vi "Dashboard Main.vi"() -> ()   [LabVIEW 2017]
uses:
  <vilib>/Rock Robotics/Network Tables/NT Read Numeric Array.vi
  <vilib>/Rock Robotics/Network Tables/NT Read Number.vi
  <vilib>/Rock Robotics/Network Tables/NT Write Boolean.vi
panel:
  out "Camera Info":cluster{"Mbps LED":bool, "Mbps":dbl, "fps":dbl} {"fps" format="%#.1g"; "Mbps" format="%#.1g"}
  in  "Camera Settings":T1={"Frame Rate"=30, "Compression"=30, "Size"=1, "DB Camera Config"=FALSE} {"Frame Rate" scale=1.0..30.0; "Compression" scale=100.0..-1.0; "Size" items=["640x480", "320x240", "160x120"]}
  in  "TCP":refnum<k5>
  out "Robot IP":string
  in  "Dashboard Tab":enum32{"Drive", "Basic", "Custom", "Variables"}(tab)
  out "Accel mins":dbl[](array[numeric])
  in  "Boolean":bool
  out "AvgY":dbl
  out "AvgX":dbl
  out "Accel maxs":dbl[](array[numeric])
  out "Accels":dbl[](array[numeric])
  out "Gyro rate":dbl
  out "Gyro":dbl
  in  "Select Auto":string(combo)="Select Autonomous ..."
  out "NT Connection":bool
  out "MotorChart R":cluster{"Numeric":dbl, "Numeric":dbl}(graph)
  out "MotorChart L":cluster{"Numeric":dbl, "Numeric":dbl}(graph)
  out "MotorSliders R":cluster{"MotorSlide1":dbl, "MotorSlide2":dbl} {"MotorSlide2" scale=-1.0..1.0 scale format="%#_2e"; "MotorSlide1" scale=-1.0..1.0 scale format="%#_2e"}
  out "MotorSliders L":cluster{"MotorSlide1":dbl, "MotorSlide2":dbl} {"MotorSlide2" scale=-1.0..1.0 scale format="%#_2e"; "MotorSlide1" scale=-1.0..1.0 scale format="%#_2e"}
  out "JS1 Z":dbl(slide) scale=-1.0..1.0 scale format="%#_2e"
  out "JS1 Graph":cluster{"X":dbl, "Y":dbl}[](graph)
  out "JS1 Buttons":T2
  out "JS2 Z":dbl(slide) scale=-1.0..1.0 scale format="%#_2e"
  out "JS2 Graph":cluster{"X":dbl, "Y":dbl}[](graph)
  out "JS2 Buttons":T2
  out "Mode":T3(ring)=enum."Auto Disabled"
  in  "DB/String 9":string
  in  "DB/String 8":string
  in  "DB/String 7":string
  in  "DB/String 6":string
  in  "DB/String 5":string
  in  "DB/String 4":string
  in  "DB/String 3":string
  in  "DB/String 2":string
  in  "DB/String 1":string
  in  "DB/String 0":string
  in  "DB/Slider 0":dbl(slide) scale=0.0..5.0
  in  "DB/Slider 1":dbl(slide) scale=0.0..5.0
  in  "DB/Slider 2":dbl(slide) scale=0.0..5.0
  in  "DB/Slider 3":dbl(slide) scale=0.0..5.0
  out "DB/LED 3":bool
  out "DB/LED 2":bool
  out "DB/LED 1":bool
  out "DB/LED 0":bool
  in  "DB/Button 3":bool
  in  "DB/Button 2":bool
  in  "DB/Button 1":bool
  in  "DB/Button 0":bool caption="New Name"
  out "Tree":string(tree)
  out "Camera Image":T4(plugin-control)
  out "Background":bool
  in  "Camera Name":string(combo)="No Camera Selection"
  # "HW"
  # "Joysticks"
  # "Drive Motors"
  # "Front"
  # "Right"
  # "Left"
  # "Back"
  # "This tab is a great place for autonomous settings and robot-specific values.\nPlace controls and indicators inside this tab and match name to\nDashboard Variables on robot. You can also delete this comment."
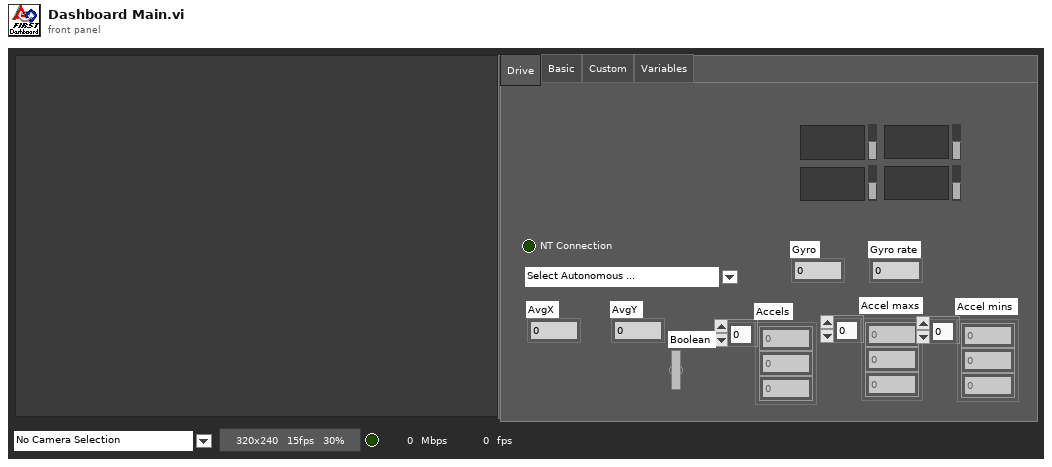
[diagram p1: front panel]
types:
  T1 = cluster{"Frame Rate":i32, "Compression":i32, "Size":u16, "DB Camera Config":bool}
  T2 = cluster{bool, bool, bool, bool, bool, bool, bool, bool, bool, bool, bool, bool}
  T3 = enum8{"Tele-Op Disabled", "Tele-Op Enabled", "Auto Disabled", "Auto Enabled", "Test Disabled", "Test Enabled", "Disconnected", "No Code", "E-Stop"}
  T4 = typedef "IMAQ Image.ctl" = refnum<image>
  T5 = cluster{"Save Path":path, "Interval (s)":dbl, "Keep":i32}
  T6 = typedef "Image Type" = u32
  T7 = cluster{"Camera Image":refnum<vi>, "Dashboard Tab":refnum<vi>, "Background":refnum<vi>, "Tree":refnum<vi>, "Camera Settings":refnum<vi>, "Camera Name":refnum<vi>, "Camera Info":refnum<vi>}
  T8 = cluster{"Error Strings":string, "Disable Counts":cluster{u16, u16}, "Rail Faults":cluster{u16, u16, u16}, "Robot IP":string, "DB Mode":u8, "Event Info":cluster{"Name":string, "Type":u8, "Number":u16, "Replay":u8}}
  T9 = cluster{"Storage":cluster{"Disk Free":u64, "RAM Block":u32, "RAM free":u32}, "CPU Utilization":cluster{"CPU % ISR":sgl, "CPU % Time Crit":sgl, "CPU % Timed Str":sgl, "CPU % High":sgl, "CPU % Above":sgl, "CPU % Normal":sgl, "CPU % Low":sgl}, "CAN":cluster{"% Bus Utilization":sgl, "Bus Off Cnt":u32, "TX_FIFO Full Cnt":u32, "Receive Error Cnt":u8, "Transmit Error Cnt":u8}, "HID":cluster{"HID Outputs":u32, "Rumble Low":u16, "Rumble High":u16}[]}
  T10 = cluster{"Status bits":cluster{"Test Mode":bool, "Autonomous":bool, "Enabled":bool, "Code Start":bool, "Brownout":bool, "Reserved 2":bool, "Reserved 3":bool, "E-Stop":bool}, "Code Trace":cluster{"Disabled":bool, "TeleOp":bool, "Auto":bool, "Test":bool}, "Controller Type":enum16{"unknown", "cRIO", "roboRio"}, "Code?":enum16{"unknown", "noCode", "code"}, "Battery V":dbl}
  T11 = cluster{"Control Bits":cluster{"TestMode":bool, "Autonomous":bool, "Enabled":bool, "FMS Present":bool, bool, bool, bool, "E-Stop":bool}, "Team Station ":u8, "Countdown":sgl, "Joystick Values":cluster{"Axes":dbl[], "Buttons":bool[], "POVs":i16[]}[]}
  T12 = cluster{"Axes":dbl[], "Buttons":bool[], "POVs":i16[]}[]
  T13 = cluster{"Axes":dbl[], "Buttons":bool[], "POVs":i16[]}
  T14 = cluster{"Buttons[0]":bool, "Buttons[1]":bool, "Buttons[2]":bool, "Buttons[3]":bool, "Buttons[4]":bool, "Buttons[5]":bool, "Buttons[6]":bool, "Buttons[7]":bool, "Buttons[8]":bool, "Buttons[9]":bool, "Buttons[10]":bool, "Buttons[11]":bool}
  T15 = cluster{"Shift":bool, "Ctrl":bool, "Alt":bool, "Cmd":bool, "Opt":bool}
  T16 = cluster{"Camera Name":string, "Camera File Name":string, "Saved DB Images Info":cluster{"Save Path":path, "Interval (s)":dbl, "Keep":i32}}
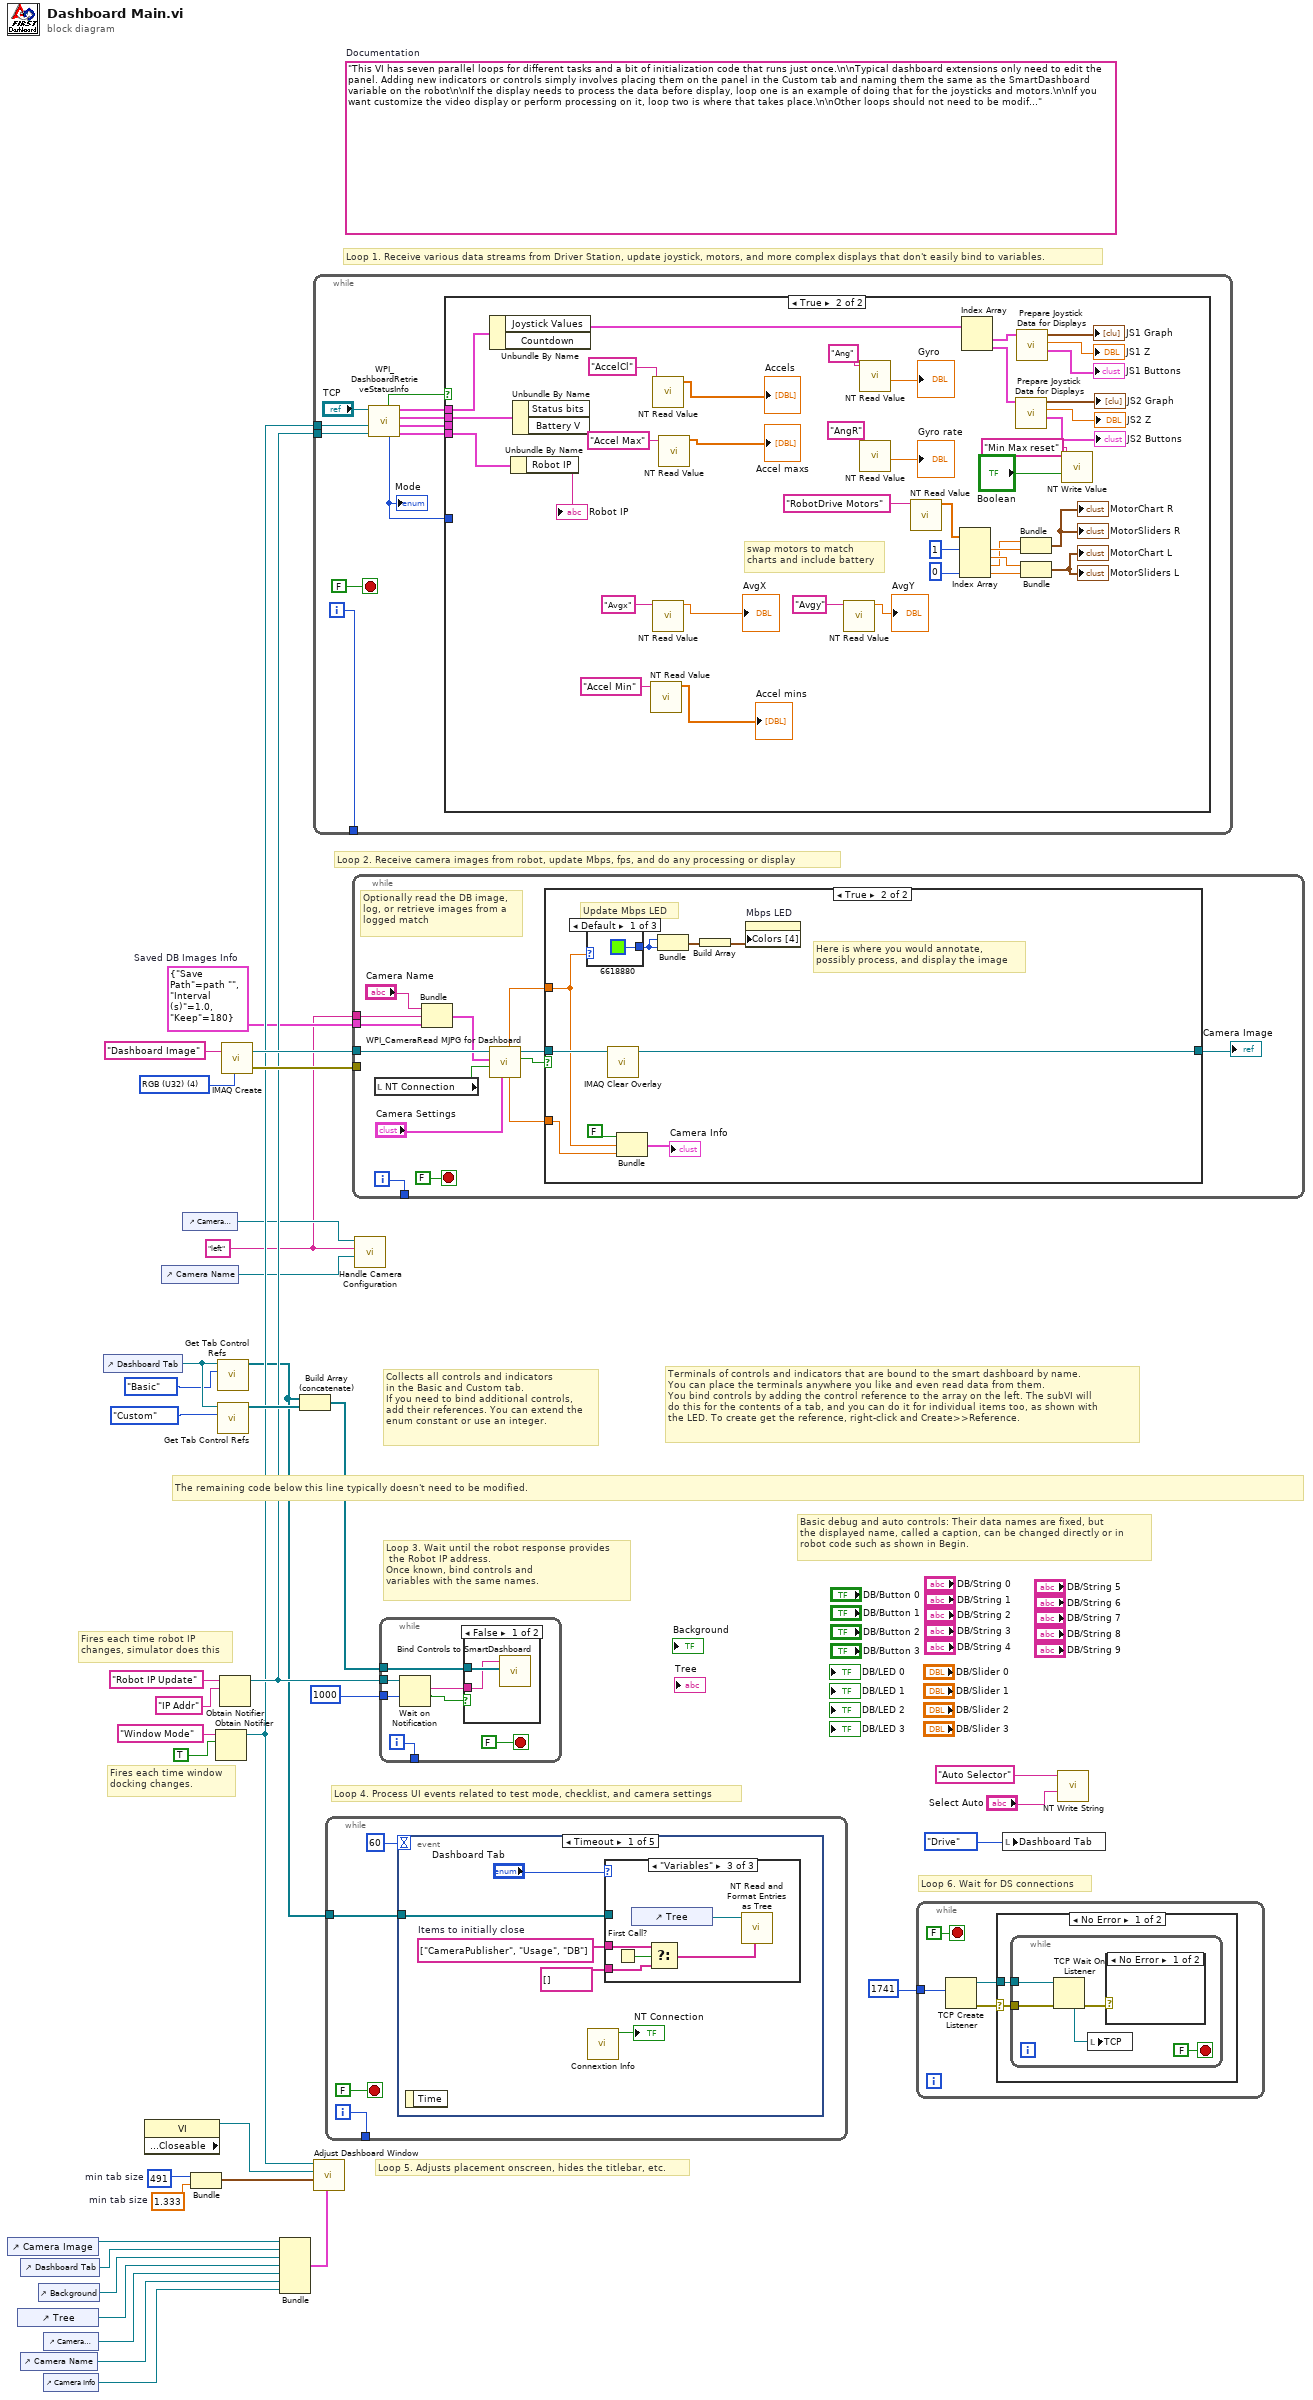
[diagram p0: block diagram]
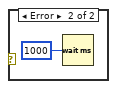
[diagram p2: hidden frame]
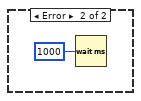
[diagram p3: hidden frame]
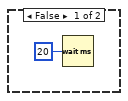
[diagram p4: hidden frame]
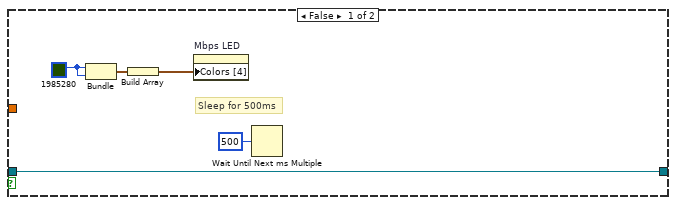
[diagram p6: hidden frame]
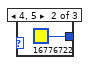
[diagram p7: hidden frame]
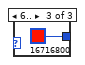
[diagram p8: hidden frame]
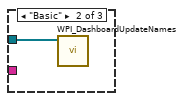
[diagram p10: hidden frame]
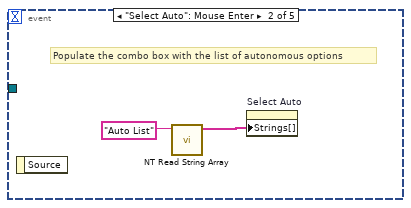
[diagram p11: hidden frame]
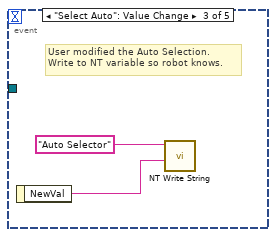
[diagram p12: hidden frame]
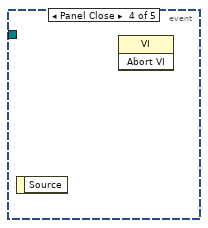
[diagram p13: hidden frame]
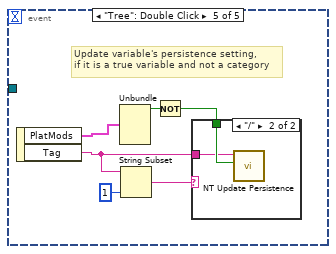
[diagram p14: hidden frame]
diagram:
  w1 = "left" ("Camera File Name")
  w2 = T5 {"Save Path"=path "", "Interval (s)"=1.0, "Keep"=180}  # Saved DB Images Info
  w22 = 491  # min tab size
  w21 = 1.333  # min tab size
  (unwired) "This VI has seven parallel loops for different tasks and a bit of initialization code that runs just once.\n\nTypical dashboard extensions only need to edit the panel. Adding new indicators or controls simply involves placing them on the panel in the Custom tab and naming them the same as the SmartDashboard variable on the robot\n\nIf the display needs to process the data before display, loop one is an example of doing that for the joysticks and motors.\n\nIf you want customize the video display or perform processing on it, loop two is where that takes place.\n\nOther loops should not need to be modified. They are pretty standard, and document the task they perform."  # Documentation
  w37 = T6 4 items=["Grayscale (U8)", "Grayscale (I16)", "Grayscale (SGL)", "Complex (CSG)", "RGB (U32)", "HSL (U32)", "RGB (U64)"] ("Image Type")
  # "Loop 6. Wait for DS connections"
  # "Basic debug and auto controls: Their data names are fixed, but\nthe displayed name, called a caption, can be changed directly or in\nrobot code such as shown in Begin."
  # "Fires each time robot IP\nchanges, simulator does this"
  # "Fires each time window\ndocking changes."
  # "Collects all controls and indicators\nin the Basic and Custom tab.\nIf you need to bind additional controls,\nadd their references. You can extend the\nenum constant or use an integer."
  # "The remaining code below this line typically doesn't need to be modified."
  # "Loop 4. Process UI events related to test mode, checklist, and camera settings"
  # "Terminals of controls and indicators that are bound to the smart dashboard by name.\nYou can place the terminals anywhere you like and even read data from them.\nYou bind controls by adding the control reference to the array on the left. The subVI will\ndo this for the contents of a tab, and you can do it for individual items too, as shown with\nthe LED. To create get the reference, right-click and Create>>Reference."
  # "Loop 3. Wait until the robot response provides\n the Robot IP address.\nOnce known, bind controls and\nvariables with the same names."
  # "Loop 5. Adjusts placement onscreen, hides the titlebar, etc."
  # "Loop 1. Receive various data streams from Driver Station, update joystick, motors, and more complex displays that don't easily bind to variables."
  # "Loop 2. Receive camera images from robot, update Mbps, fps, and do any processing or display"
  n1 = control-ref of="Camera Image"() -> (w24:refnum<vi>)
  n2 = control-ref of="Tree"() -> (w8:refnum<vi>)
  n3 = control-ref of="Dashboard Tab"() -> (w23:refnum<vi>)
  n4 = control-ref of="Camera Name"() -> (w6:refnum<vi>)
  n5 = control-ref of="Background"() -> (w19:refnum<vi>)
  n6 = control-ref of="Camera Settings"() -> (w7:refnum<vi>)
  n7 = control-ref of="Camera Info"() -> (w5:refnum<vi>)
  n8 = control-ref of="Dashboard Tab"() -> (w27:refnum<vi>)
  n9 = property class="VI" props=["Front Panel.Closeable"]() -> (reference out=w28:refnum<vi>)  [unwired: 2 in, 2 out]
  n10 = control-ref of="Camera Name"() -> (w12:refnum<vi>)
  n11 = control-ref of="Camera Settings"() -> (w13:refnum<vi>)
  n12 = Bundle("min tab size"=w22, "min tab size"=w21) -> (w20:cluster{"min tab size":i32, "min tab size":dbl})  [unwired: 1 in]
  n13 = Obtain Notifier(name (unnamed)="Window Mode", notification data type=TRUE) -> (notifier out=w16:refnum<notifier>)  [unwired: 2 in, 2 out]
  n14 = call <vilib>:"Get Tab Control Refs.vi"("Page Index"=enum32{"Drive", "Basic", "Custom", "Variables"}."Basic" ("Dashboard Tab"), "TabControl in"=w27) -> ("ControlsOnPage"=w11:refnum<vi>[])  [unwired: 9 in]
  n15 = call <vilib>:"Get Tab Control Refs.vi"("Page Index"=enum32{"Drive", "Basic", "Custom", "Variables"}."Custom" ("Dashboard Tab"), "TabControl in"=w27) -> ("ControlsOnPage"=w26:refnum<vi>[])  [unwired: 9 in]
  n16 = Obtain Notifier(name (unnamed)="Robot IP Update", notification data type="IP Addr" ("name (unnamed)")) -> (notifier out=w17:refnum<notifier>)  [unwired: 2 in, 2 out]
  n17 = call "IMAQ Create"("Image Name"="Dashboard Image", "Image Type"=w37) -> ("New Image"=w35:T4, "error out"=w34:errorcluster)  [unwired: 2 in, 1 out]
  n18 = Bundle("Camera Image"=w24, "Dashboard Tab"=w23, "Background"=w19, "Tree"=w8, "Camera Settings"=w7, "Camera Name"=w6, "Camera Info"=w5) -> (w18:T7)  [unwired: 1 in]
  n19 = Build Array (concatenate)(w11, w26) -> (w25:refnum<vi>[])
  n20 = while {
    tunnel: [w47] -> _
    tunnel: w17 -> [w41]
    tunnel: w16 -> [w38]
    i -> [w47]
    stop <- FALSE stop-if-true
    n21 = call <vilib>:"WPI_DashboardRetrieveStatusInfo.vi"("Binding Refnum"=w41, "Window Mode Notifier"=w38, "TCP Cnx"="TCP") -> ("Power and Errors"=w42:T8, "Robot Metrics"=w45:T9, "Status Info"=w46:T10, "Control Info"=w43:T11, "Robot Mode"=w40:T3, "Process?"=w44:bool)  [unwired: 3 in]
    "Mode" <- w40
    n22 = case shown="True" w44 {
      tunnel: w46 -> [_ w88]
      tunnel: w45 -> [_ _]
      tunnel: w43 -> [_ w87]
      tunnel: w42 -> [_ w86]
      tunnel: w40 -> [_ _]
      frame False {
        n23 = Wait (ms)(milliseconds to wait=u32 20) -> ()  [unwired: 1 out]
      }
      frame True {
        # "swap motors to match\ncharts and include battery"
        n24 = Unbundle By Name(w87) -> ("Joystick Values"=w77:T12)  [unwired: 1 out]
        n25 = Unbundle By Name(w86) -> ("Robot IP"=→"Robot IP":string)
        n26 = Unbundle By Name(w88) -> ()  [unwired: 2 out]
        n27 = call-poly <vilib>:"NT Read Value.vi"("Name"="Accel Min") -> ("Numeric Array"=→"Accel mins":dbl[])  [unwired: 9 in, 1 out]
        n28 = call-poly <vilib>:"NT Read Value.vi"("Name"="AccelCl") -> ("Numeric Array"=→"Accels":dbl[])  [unwired: 9 in, 1 out]
        n29 = call-poly <vilib>:"NT Read Value.vi"("Name"="Avgx") -> ("Numeric"=→"AvgX":dbl)  [unwired: 9 in, 1 out]
        n30 = call-poly <vilib>:"NT Read Value.vi"("Name"="Accel Max") -> ("Numeric Array"=→"Accel maxs":dbl[])  [unwired: 9 in, 1 out]
        n31 = call-poly <vilib>:"NT Read Value.vi"("Name"="Avgy") -> ("Numeric"=→"AvgY":dbl)  [unwired: 9 in, 1 out]
        n32 = call-poly <vilib>:"NT Read Value.vi"("Name"="Ang") -> ("Numeric"=→"Gyro":dbl)  [unwired: 9 in, 1 out]
        n33 = call-poly <vilib>:"NT Read Value.vi"("Name"="AngR") -> ("Numeric"=→"Gyro rate":dbl)  [unwired: 9 in, 1 out]
        n34 = call-poly <vilib>:"NT Read Value.vi"("Name"="RobotDrive Motors") -> ("Numeric Array"=w67:dbl[])  [unwired: 9 in, 1 out]
        n35 = Index Array(array=w67, index #1=1, index #4=0) -> (element #1=w81:dbl, element #2=w82:dbl, element #3=w80:dbl, element #4=w85:dbl)  [unwired: 2 in]
        n36 = Index Array(array=w77) -> (element #1=w76:T13, element #2=w72:T13)  [unwired: 2 in]
        n37 = call "Prepare Joystick Data for Displays.vi"("Joystick Values"=w72) -> ("Buttons"=→"JS2 Buttons":T14, "Z Axis"=→"JS2 Z":dbl, "Cartesian Data"=→"JS2 Graph":cluster{"X axis":dbl, "X axis":dbl}[])  [unwired: 8 in]
        n38 = call "Prepare Joystick Data for Displays.vi"("Joystick Values"=w76) -> ("Buttons"=→"JS1 Buttons":T14, "Z Axis"=→"JS1 Z":dbl, "Cartesian Data"=→"JS1 Graph":cluster{"X axis":dbl, "X axis":dbl}[])  [unwired: 8 in]
        n39 = Bundle("Numeric"=w80, "Numeric"=w81) -> (→"MotorChart R" →"MotorSliders R":cluster{"Numeric":dbl, "Numeric":dbl})  [unwired: 1 in]
        n40 = Bundle("Numeric"=w82, "Numeric"=w85) -> (→"MotorChart L" →"MotorSliders L":cluster{"Numeric":dbl, "Numeric":dbl})  [unwired: 1 in]
        n41 = call-poly <vilib>:"NT Write Value.vi"("Boolean"="Boolean", "Name"="Min Max reset") -> ()  [unwired: 9 in, 1 out]
      }
    }
  }
  n42 = call "Adjust Dashboard Window.vi"("Sizing Refnums"=w18, "Size Constraints"=w20, "VI"=w28, "WIn Mode"=w16) -> ()  [unwired: 8 in]
  n43 = while {
    tunnel: [w90] -> _
    tunnel: w11 -> [w89]
    i -> [w90]
    stop <- FALSE stop-if-true
    n44 = event shown="[0] Timeout" {
      selector: _ -> [_ _ _ _ _]
      dyn-events: _ -> [_ _ _ _ _]
      timeout: u32 60 ("milliseconds to wait") -> [_ _ _ _ _]
      tunnel: w89 -> [w95 _ _ _ _]
      event Timeout {
        w94 = string[] ["CameraPublisher", "Usage", "DB"]  # Items to initially close
        n45 = event-data() -> ()  [unwired: 1 in, 1 out]
        n46 = call <vilib>:"Connextion Info.vi"() -> ("Connected"=→"NT Connection":bool)  [unwired: 10 in, 1 out]
        n47 = case shown="\"Variables\"" "Dashboard Tab" {
          tunnel: w95 -> [_ w98 _]
          tunnel: w94 -> [_ _ w101]
          tunnel: string[] [] -> [_ _ w100]
          frame "Custom", Default {
          }
          frame "Basic" {
            n48 = call <vilib>:"WPI_DashboardUpdateNames.vi"("Controls on Tab"=w98) -> ()  [unwired: 11 in]
          }
          frame "Variables" {
            n49 = First Call?() -> (First Call?: T/F=w102:bool)
            n50 = control-ref of="Tree"() -> (w103:refnum<vi>)
            n51 = Select(t=w101, s=w102, f=w100) -> (s? t:f=w99:string[])
            n52 = call <vilib>:"NT Read and Format Entries as Tree.vi"("Tags to  Close"=w99, "Tree Refnum"=w103) -> ()  [unwired: 8 in, 2 out]
          }
        }
      }
      event "Select Auto": Mouse Enter {
        # "Populate the combo box with the list of autonomous options"
        n53 = event-data() -> ()  [unwired: 1 in, 1 out]
        n54 = call <vilib>:"NT Read String Array.vi"("Name"="Auto List") -> ("String Array"=w104:string[])  [unwired: 9 in, 1 out]
        n55 = property on="Select Auto" class="CmbBox"("Strings[]"=w104) -> ()  [unwired: 2 in, 2 out]
      }
      event "Select Auto": Value Change {
        # "User modified the Auto Selection.\nWrite to NT variable so robot knows."
        n56 = event-data() -> ("NewVal"=w106:string)  [unwired: 1 in]
        n57 = call <vilib>:"NT Write String.vi"("String"=w106, "Name"="Auto Selector") -> ()  [unwired: 9 in, 1 out]
      }
      event Panel Close {
        n58 = event-data() -> ()  [unwired: 1 in, 1 out]
        n59 = invoke class="VI" method="Abort VI"() -> ()  [unwired: 3 in, 3 out]
      }
      event "Tree": Double Click {
        # "Update variable's persistence setting,\nif it is a true variable and not a category"
        n60 = event-data() -> ("PlatMods"=w109:T15, "Tag"=w108:string)  [unwired: 1 in]
        n61 = Unbundle(w109) -> ("Shift"=w113:bool)  [unwired: 4 out]
        n62 = String Subset(string=w108, length (rest)=1 ("length (rest)")) -> (substring=w110:string)  [unwired: 1 in]
        n63 = Not(x=w113) -> (.not. x?=w112:bool)
        n64 = case shown="\"/\"" w110 {
          tunnel: w112 -> [_ w115]
          tunnel: w108 -> [_ w114]
          frame Default {
          }
          frame "/" {
            n65 = call <vilib>:"NT Update Persistence.vi"("Persistence"=w115, "Name"=w114) -> ()  [unwired: 9 in, 1 out]
          }
        }
      }
    }
  }
  n66 = while {
    tunnel: w35 -> [w127]
    tunnel: w34 -> [_]
    tunnel: [w128] -> _
    tunnel: w2 -> [w119]
    tunnel: w1 -> [w116]
    i -> [w128]
    stop <- FALSE stop-if-true
    # "Optionally read the DB image,\nlog, or retrieve images from a\nlogged match"
    n67 = local read "NT Connection"() -> (w120:bool)
    n68 = Bundle("Camera Name"="Camera Name", "Camera File Name"=w116, "Saved DB Images Info"=w119) -> (w118:T16)  [unwired: 1 in]
    n69 = call <vilib>:"WPI_CameraRead MJPG for Dashboard.vi"("Camera Settings"="Camera Settings", "NT Connection"=w120, "Capture Info"=w118, "Refnum in"=w127) -> ("Active"=w125:bool, "Refnum out"=w126:T4, "FPS"=w124:dbl, "Bandwidth (Mbps)"=w123:dbl)  [unwired: 4 in]
    n70 = case shown="True" w125 {
      tunnel: w126 -> [w130 w141]
      tunnel: w123 -> [_ w138]
      tunnel: w124 -> [_ w139]
      tunnel: [w130 w135] -> w121
      frame False {
        w132 = u32 1985280 ("Color Box")
        # "Sleep for 500ms"
        n71 = Bundle("Color Box"=w132, "Color Box"=w132) -> (w133:cluster{"Color Box":u32, "Color Box":u32})  [unwired: 1 out]
        n72 = Build Array(w133) -> (w131:cluster{"Color Box":u32, "Color Box":u32}[])
        n73 = property on="Mbps LED" class="Bool (strict)"("Colors [4]"=w131) -> ()  [unwired: 2 in, 2 out]
        n74 = Wait Until Next ms Multiple(millisecond multiple=u32 500) -> ()  [unwired: 1 out]
      }
      frame True {
        # "Here is where you would annotate,\npossibly process, and display the image"
        # "Update Mbps LED"
        n75 = case shown="Default" w138 {
          tunnel: [u32 6618880 ("Color Box") u32 16776722 ("Color Box") u32 16716800 ("Color Box")] -> w142
          frame Default {
          }
          frame 4, 5 {
          }
          frame 6.. {
          }
        }
        n76 = call "IMAQ Clear Overlay"("Image"=w141) -> ("Image Out"=w135:T4)  [unwired: 2 in, 8 out]
        n77 = Bundle(FALSE, "Bandwidth (Mbps)"=w138, "FPS"=w139) -> (→"Camera Info":cluster{bool, "Bandwidth (Mbps)":dbl, "FPS":dbl})  [unwired: 1 in]
        n78 = Bundle("Color Box"=w142, "Color Box"=w142) -> (w143:cluster{"Color Box":u32, "Color Box":u32})  [unwired: 1 out]
        n79 = Build Array(w143) -> (w140:cluster{"Color Box":u32, "Color Box":u32}[])
        n80 = property on="Mbps LED" class="Bool (strict)"("Colors [4]"=w140) -> ()  [unwired: 2 in, 2 out]
      }
    }
    "Camera Image" <- w121
  }
  n81 = call "Handle Camera Configuration.vi"("CameraNameRef"=w12, "Camera File Name"=w1, "ClusterRef"=w13) -> ()  [unwired: 9 in]
  n82 = while {
    tunnel: w25 -> [w153]
    tunnel: w17 -> [w151]
    tunnel: [w149] -> _
    tunnel: u32 1000 ("milliseconds to wait") -> [w148]
    i -> [w149]
    stop <- FALSE stop-if-true
    n83 = Wait on Notification(notifier=w151, timeout in ms (-1)=w148) -> (notification=w150:string, timed out?=w147:bool)  [unwired: 2 in, 2 out]
    n84 = case shown="False" w147 {
      tunnel: w153 -> [w155 _]
      tunnel: w150 -> [w154 _]
      frame False {
        n85 = call <vilib>:"Bind Controls to SmartDashboard.vi"("Bound Control Refs"=w155, "Server IP Address"=w154) -> ()  [unwired: 10 in]
      }
      frame True {
      }
    }
  }
  n86 = while {
    tunnel: u16 1741 ("timeout ms (25000)") -> [w157]
    stop <- FALSE stop-if-true
    n87 = TCP Create Listener(10:w157) -> (0:w156:errorcluster, 3:w158:refnum<k5>)  [unwired: 4 in, 1 out]
    n88 = case shown="No Error" w156 {
      selector: w156 -> [w160 _]
      tunnel: w158 -> [w161 _]
      frame No Error {
        n89 = while {
          tunnel: w161 -> [w164]
          tunnel: w160 -> [w163]
          stop <- FALSE stop-if-true
          n90 = TCP Wait On Listener(8:w163, 11:w164) -> (0:w165:errorcluster, 4:w166:refnum<k5>)  [unwired: 2 in, 3 out]
          n91 = local write "TCP"(w166) -> ()
          n92 = case shown="No Error" w165 {
            frame No Error {
            }
            frame Error {
              n93 = Wait (ms)(milliseconds to wait=u32 1000) -> ()  [unwired: 1 out]
            }
          }
        }
      }
      frame Error {
        n94 = Wait (ms)(milliseconds to wait=u32 1000) -> ()  [unwired: 1 out]
      }
    }
  }
  n95 = local write "Dashboard Tab"(enum32{"Drive", "Basic", "Custom", "Variables"}."Drive" ("Dashboard Tab")) -> ()
  n96 = call <vilib>:"NT Write String.vi"("String"="Select Auto", "Name"="Auto Selector") -> ()  [unwired: 9 in, 1 out]
